vi "Write new ixon op mode.vi"(8 "error in (no error)":errorcluster, 9 "new operation mode":T1, 10 "new ixon op mode":T2={"EM_MODE"=20, "EM_GAIN"=0, "FRAME_TRANSFER"=FALSE}, 11 "Sim_Ixon_Ultra in":refnum<class "Sim_Ixon_Ultra.lvclass">) -> (0 "error out":errorcluster, 3 "Sim_Ixon_Ultra out":refnum<class "Sim_Ixon_Ultra.lvclass">)   [LabVIEW 2018, in "Sim_Ixon_Ultra.lvclass"]
uses:
  Sim_Ixon_Ultra.lvclass
  C:/Users/Denis/Desktop/S4ACS/S4ACS/Simulated_CCD_Camera/Simulated Camera.lvclass
  Sim_Ixon_Ultra.lvclass/Sim_Ixon_Ultra.ctl
  Simulated_CCD_Camera/Simulated Camera.lvclass
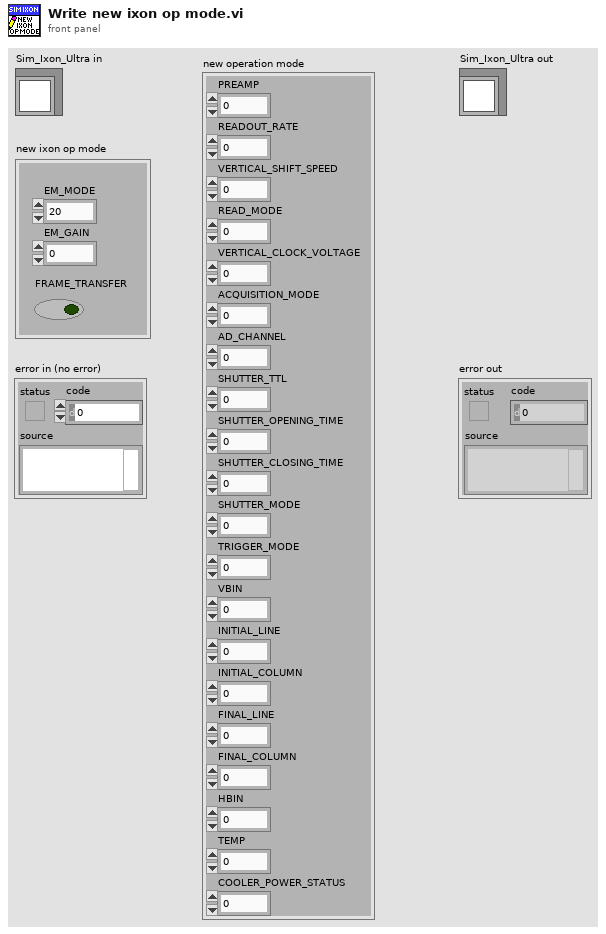
[diagram p1: front panel]
types:
  T1 = cluster{"PREAMP":u16, "READOUT_RATE":u16, "VERTICAL_SHIFT_SPEED":u16, "READ_MODE":u16, "VERTICAL_CLOCK_VOLTAGE":u16, "ACQUISITION_MODE":u16, "AD_CHANNEL":u16, "SHUTTER_TTL":u16, "SHUTTER_OPENING_TIME":u16, "SHUTTER_CLOSING_TIME":u16, "SHUTTER_MODE":u16, "TRIGGER_MODE":u16, "VBIN":u16, "INITIAL_LINE":u16, "INITIAL_COLUMN":u16, "FINAL_LINE":u16, "FINAL_COLUMN":u16, "HBIN":u16, "TEMP":u16, "COOLER_POWER_STATUS":u16}
  T2 = cluster{"EM_MODE":u16, "EM_GAIN":u16, "FRAME_TRANSFER":bool}
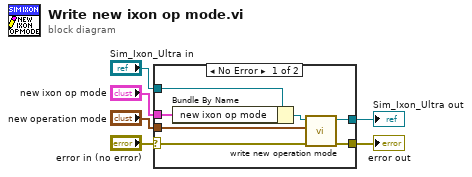
[diagram p0: block diagram]
diagram:
  n1 = case shown="No Error" "error in (no error)" {
    selector: "error in (no error)" -> [w9 w14]
    tunnel: [w8 w14] -> w5
    tunnel: [w10 w15] -> w3
    tunnel: "Sim_Ixon_Ultra in" -> [w13 w15]
    tunnel: "new ixon op mode" -> [w12 _]
    tunnel: "new operation mode" -> [w7 _]
    frame No Error {
      n2 = Bundle By Name(cluster=w13, "new ixon op mode"=w12) -> (w11:refnum<class "Sim_Ixon_Ultra.lvclass">)
      n3 = call "write new operation mode.vi"("error in (no error)"=w9, "new operation mode"=w7, "CCDCamera in"=w11) -> ("error out"=w8:errorcluster, "CCDCamera out"=w10:refnum<class "Sim_Ixon_Ultra.lvclass">)  [unwired: 7 in]
    }
    frame Error {
    }
  }
  "error out" <- w5
  "Sim_Ixon_Ultra out" <- w3
